vi "Laser power controller.vi"(8 "error in (no error)":errorcluster, 11 "Laser Power Controller in":refnum<class "Laser Power Controller.lvclass">) -> (0 "error out":errorcluster, 3 "Laser Power Controller out":refnum<class "Laser Power Controller.lvclass">)   [LabVIEW 2009, in "Laser Power Controller.lvclass"]
uses:
  Laser Power Controller.lvclass
  Global/GPIB Numbers.vi
panel:
  out "Status":string
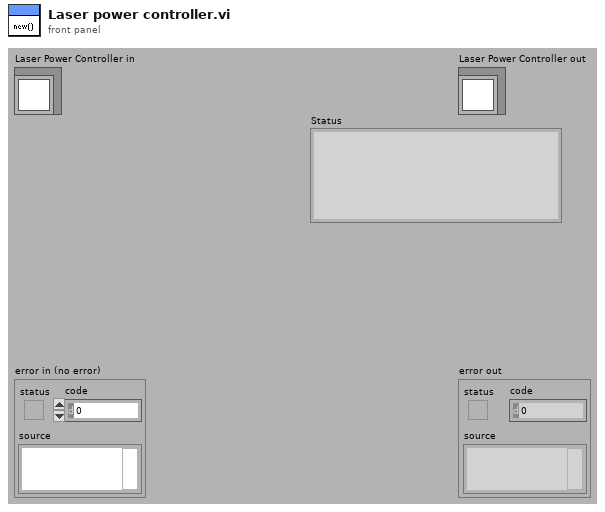
[diagram p1: front panel]
types:
  T1 = typedef "GPIB Type Def.ctl" = cluster{"Name":string, "bus":dbl, "GPIB":dbl, "GPIB as string":string, "byte":i32, "VISA Resource Name":refnum<visa-resource-name>}
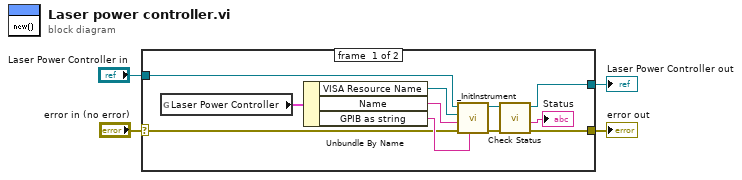
[diagram p0: block diagram]
diagram:
  n1 = case shown="No Error" "error in (no error)" {
    selector: "error in (no error)" -> [w10 w17]
    tunnel: [w6 w17] -> w3
    tunnel: [w8 w16] -> w1
    tunnel: "Laser Power Controller in" -> [w14 w16]
    frame #0 {
      n2 = global read "GPIB Numbers.vi" "Laser Power Controller"() -> (w15:T1)
      n3 = Unbundle By Name(w15) -> ("VISA Resource Name"=w13:refnum<visa-resource-name>, "Name"=w12:string, "GPIB as string"=w11:string)
      n4 = call-dynamic "_InitInstrument.vi"("GPIB as string"=w11, "error in (no error)"=w10, "Name"=w12, "VISA Resource Name"=w13, "Instrument in"=w14) -> ("error out"=w7:errorcluster, "Instrument out"=w9:refnum<class "Laser Power Controller.lvclass">)  [unwired: 1 in, 4 out]
      n5 = call-dynamic "Check Status.vi"("error in (no error)"=w7, "Laser Power Controller in"=w9) -> ("error out"=w6:errorcluster, "Status"=→"Status":string, "Laser Power Controller out"=w8:refnum<class "Laser Power Controller.lvclass">)  [unwired: 6 in, 1 out]
    }
    frame #1 {
    }
  }
  "error out" <- w3
  "Laser Power Controller out" <- w1
